vi "Open Subscriber.vi"(7 "EventLogging":refnum<class "EventLoggingService.lvclass">, 9 "Telemetry Config":T4, 10 "Subscription":T3, 11 "IP Resolver":refnum<class "IP Resolver.lvclass">) -> (0 "error out":errorcluster, 3 "UDP":refnum<k16>, 5 "Subscription Loop Data":T1)   [LabVIEW 2020, in "Vecto.lvlib" / "RemoteDataService.lvclass"]
uses:
  RemoteDataService.lvclass
  RemoteDataService.lvclass/RemoteDataService.ctl
  proto/UdpPayload/UdpPayload.lvlib
  proto/UdpPayload/Data.ctl
  Group/Group.lvclass
  SubscribedDataHandler/SubscribedDataHandler.lvclass
  Subscription Group Info.ctl
  Subscription Loop Data.ctl
  EventLoggingService/EventLoggingService.lvclass
  Event Level.ctl
  Vecto.lvlib
  <vilib>/Utility/tcp.llb/UDP Multicast Read-Only Open.vi
  IP Resolver/IP Resolver.lvclass
  VectoConfig/Telemetry Routing.ctl
  VectoConfig/VectoConfig.lvlib
  VectoConfig/Endpoint.ctl
  VectoConfig/Telemetry Config.ctl
  Subscription.ctl
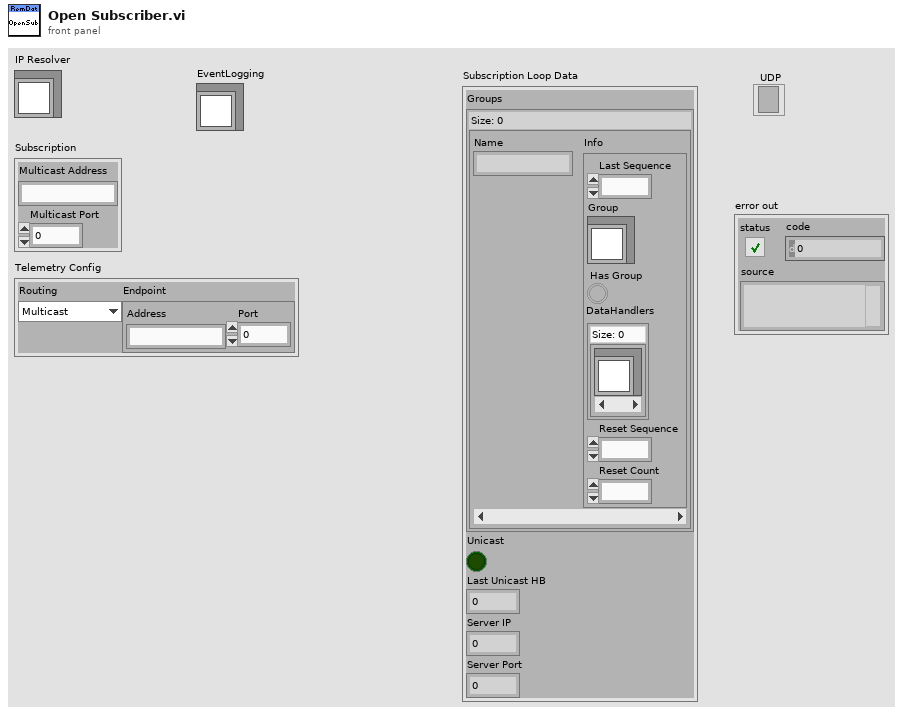
[diagram p1: front panel]
types:
  T1 = typedef "Vecto.lvlib/RemoteDataService.lvclass/Subscription Loop Data.ctl" = cluster{"Groups":map{string, T2}, "Unicast":bool, "Last Unicast HB":dbl, "Server IP":u32, "Server Port":u16}
  T2 = typedef "Vecto.lvlib/RemoteDataService.lvclass/Subscription Group Info.ctl" = cluster{"Last Sequence":u32, "Group":refnum<class "Group.lvclass">, "Has Group":bool, "DataHandlers":set{refnum<class "SubscribedDataHandler.lvclass">}, "Reset Sequence":u32, "Reset Count":u32}
  T3 = typedef "Vecto.lvlib/RemoteDataService.lvclass/Subscription.ctl" = cluster{"Multicast Address":string, "Multicast Port":u16}
  T4 = typedef "VectoConfig.lvlib/Telemetry Config.ctl" = cluster{"Routing":T5, "Endpoint":T6}
  T5 = typedef "VectoConfig.lvlib/Telemetry Routing.ctl" = enum16{"Multicast", "Unicast"}
  T6 = typedef "VectoConfig.lvlib/Endpoint.ctl" = cluster{"Address":string, "Port":u16}
  T7 = typedef "Vecto.lvlib/Event Level.ctl" = enum16{"Debug", "Info", "Warning", "Error"}
  T8 = typedef "UdpPayload.lvlib/Data.ctl" = cluster{"source_id":u32, "sequence":u32, "timestamp":i64, "type":string, "payload":u8[]}
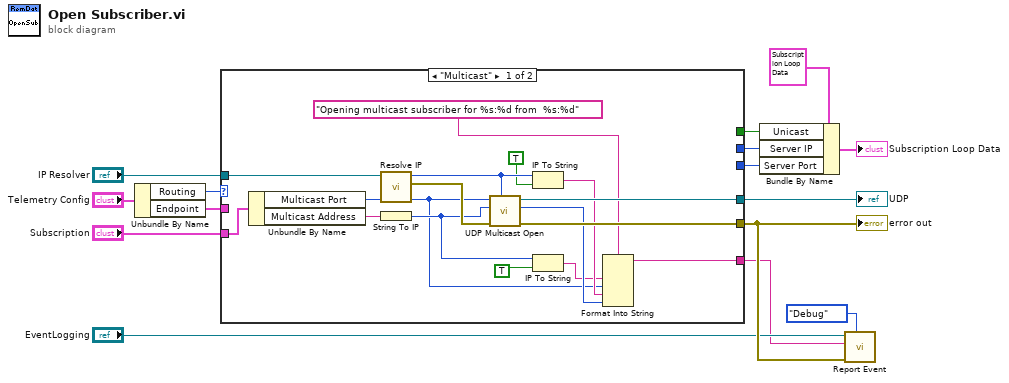
[diagram p0: block diagram]
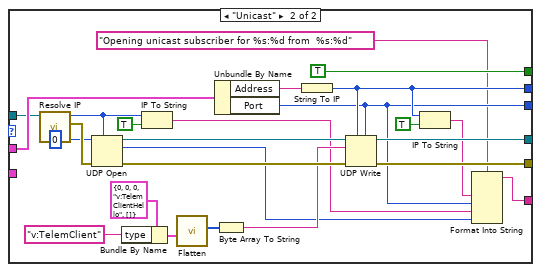
[diagram p2: hidden frame]
diagram:
  n1 = Unbundle By Name("Telemetry Config") -> ("Routing"=w12:T5, "Endpoint"=w9:T6)
  n2 = case shown="\"Multicast\"" w12 {
    tunnel: [w30 w49] -> w11
    tunnel: [w29 w51] -> w15
    tunnel: "IP Resolver" -> [w28 w33]
    tunnel: "Subscription" -> [w26 _]
    tunnel: w9 -> [_ w53]
    tunnel: [_ w38] -> w6
    tunnel: [_ w36] -> w5
    tunnel: [_ TRUE ("Unicast")] -> w4
    tunnel: [w16 w35] -> w1
    frame "Multicast" {
      n3 = Unbundle By Name(w26) -> ("Multicast Port"=w17:u16, "Multicast Address"=w27:string)
      n4 = call "Resolve IP.vi"("IP Resolver in"=w28) -> ("error out"=w31:errorcluster, "U32 Address"=w24:u32)  [unwired: 9 in]
      n5 = String To IP(1:w27) -> (0:w18:u32)
      n6 = call-poly <vilib>:"UDP Multicast Open.vi"("net address"=w24, "error in (no error)"=w31, "multicast addr"=w18, "port"=w17) -> ("error out"=w29:errorcluster, "port out"=w21:u16, "connection ID"=w30:refnum<k16>)  [unwired: 5 in]
      n7 = IP To String(1:TRUE ("dot notation? (F)"), 2:w24) -> (0:w22:string)
      n8 = IP To String(1:TRUE ("dot notation? (F)"), 2:w18) -> (0:w19:string)
      n9 = Format Into String(format string="Opening multicast subscriber for %s:%d from  %s:%d", w19, w17, w22, w21) -> (resulting string=w16:string)  [unwired: 2 in, 1 out]
    }
    frame "Unicast" {
      n10 = call "Resolve IP.vi"("IP Resolver in"=w33) -> ("error out"=w56:errorcluster, "U32 Address"=w32:u32)  [unwired: 9 in]
      n11 = UDP Open(7:w32, 8:w56, 11:u16 0 ("port")) -> (port=w50:refnum<k16>, 0:w55:errorcluster, 2:w40:u16)  [unwired: 2 in]
      n12 = Bundle By Name(cluster=T8 {"source_id"=0, "sequence"=0, "timestamp"=0, "type"="v:TelemClientHello", "payload"=[]} ("Data"), "type"="v:TelemClient") -> (w45:T8)
      n13 = IP To String(1:TRUE ("dot notation? (F)"), 2:w32) -> (0:w41:string)
      n14 = call "Flatten.vi"("Data"=w45) -> ("Buffer"=w48:u8[])  [unwired: 9 in, 1 out]
      n15 = Unbundle By Name(w53) -> ("Address"=w46:string, "Port"=w36:u16)
      n16 = Byte Array To String(unsigned byte array=w48) -> (string=w47:string)
      n17 = String To IP(1:w46) -> (0:w38:u32)
      n18 = UDP Write(address=w38, port or service name=w36, connection ID=w50, data in=w47, 8:w55) -> (error out=w51:errorcluster, 3:w49:refnum<k16>)  [unwired: 1 in]
      n19 = IP To String(1:TRUE ("dot notation? (F)"), 2:w38) -> (0:w37:string)
      n20 = Format Into String(format string="Opening unicast subscriber for %s:%d from  %s:%d", w37, w36, w41, w40) -> (resulting string=w35:string)  [unwired: 2 in, 1 out]
    }
  }
  "UDP" <- w11
  "error out" <- w15
  n21 = Bundle By Name(cluster=T1 {"Groups"={}, "Unicast"=FALSE, "Last Unicast HB"=0.0, "Server IP"=0, "Server Port"=0} ("Subscription Loop Data"), "Unicast"=w4, "Server IP"=w6, "Server Port"=w5) -> (→"Subscription Loop Data":T1)
  n22 = call "Report Event.vi"("Event Level (Info)"=Event_Level."Debug", "error in (no error)"=w15, "Message"=w1, "EventLoggingService in"="EventLogging") -> ()  [unwired: 6 in, 2 out]
